vi "dfd_FXP Simu with State.vi"(5 "input range":dbl, 6 "state in":dbl[](array[numeric]) format="%.2f", 7 "input selector":enum16{"FXP", "Integer", "Double"}(ring), 8 "error in (no error)":errorcluster, 9 "filtering statistics in":T3(array[cluster]) {"statistics information"."min value" format="%.2f"; "statistics information"."max value" format="%.2f"; "Quantizer Source" items=["Coefficients a/k"=0, "Coefficients b/v"=7, "Input"=1, "Output"=2, "Multiplicand"=3, "Product"=4, "Sum"=5, "Delay"=6]}, 10 "filter":T4 {"mSRate_QSettings"."source" items=["Coef a/k"=0, "Coef b/v"=7, "Input"=1, "Output"=2, "Multiplicand"=3, "Product"=4, "Sum"=5, "Delay"=6, "Gain"=8]}, 11 "signal in":dbl[](array[numeric])) -> (0 "error out":errorcluster, 1 "filtering statistics out":T3(array[cluster]) {"statistics information"."min value" format="%.2f"; "statistics information"."max value" format="%.2f"; "Quantizer Source" items=["Coefficients a/k"=0, "Coefficients b/v"=7, "Input"=1, "Output"=2, "Multiplicand"=3, "Product"=4, "Sum"=5, "Delay"=6]}, 2 "integer signal out":i32[](array[numeric]), 3 "DBL signal out":dbl[](array[numeric]), 4 "state out":dbl[](array[numeric]) format="%.2f")   [LabVIEW 2017, in "NI_DigFilter_FXP.lvlib"]
uses:
  <vilib>/addons/Digital Filter Design/NI_DigFilter_FXP.lvlib
  <vilib>/addons/Digital Filter Design/_Objects.llb/DFD Filter Obj.ctl
  <vilib>/addons/Digital Filter Design/_Objects.llb/DFD Filter Coef.ctl
  <vilib>/addons/Digital Filter Design/_Objects.llb/DFD Filter Structure Type Selector.ctl
  <vilib>/addons/Digital Filter Design/_Objects.llb/dfd_Internal Quantization Settings.ctl
  <vilib>/addons/Digital Filter Design/_Objects.llb/dfd_Internal Quantization Srcs.ctl
  <vilib>/addons/Digital Filter Design/_Objects.llb/DFD Coef Norm Type.ctl
  <vilib>/addons/Digital Filter Design/_Objects.llb/DFD Quantization Sources.ctl
  <vilib>/addons/Digital Filter Design/_Objects.llb/DFD FXP Statistics Data.ctl
  <vilib>/addons/Digital Filter Design/FXPLib.llb/DFD FXP to I32 (vector).vi
  <vilib>/addons/Digital Filter Design/NI_DigFilterLicensed.lvlib
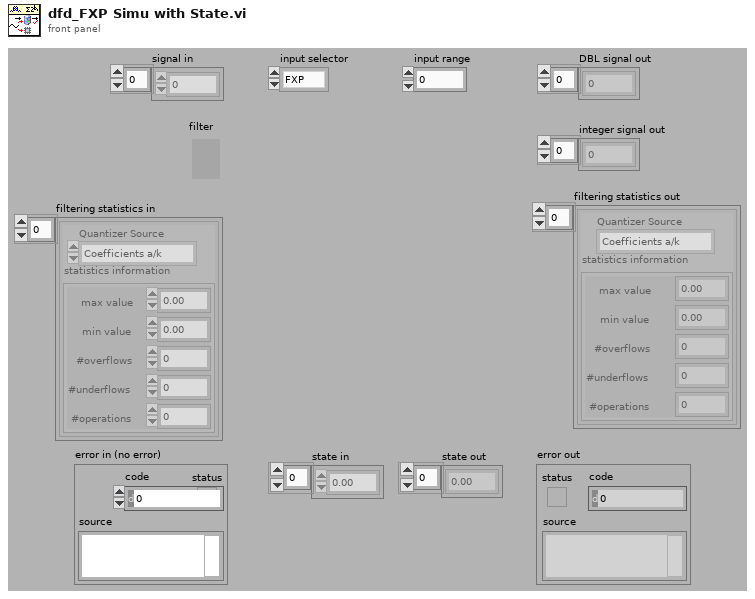
[diagram p1: front panel]
types:
  T1 = typedef "NI_DigFilterLicensed.lvlib/DFD Quantization Sources.ctl" = u16
  T2 = typedef "NI_DigFilterLicensed.lvlib/DFD FXP Statistics Data.ctl" = cluster{"max value":ext, "min value":ext, "#overflows":i32, "#underflows":i32, "#operations":i32}
  T3 = cluster{"Quantizer Source":T1, "statistics information":T2}[]
  T4 = typedef "NI_DigFilterLicensed.lvlib/DFD Filter Obj.ctl" = cluster{"mSRate_Fs":dbl, "mSRate_Version":string, "mSRate_Comments":string, "mSRate_OrgCoef":T5, "mSRate_CurCoef":T5, "mSRate_Quantized?":bool, "mSRate_QCoef":T5, "mSRate_QSettings":T7[], "mSRate_Order":i32, "mSRate_Scaling":cluster{"mSRate_ScaleByPowerOf2?":bool, "mSRate_ScaleType":T9}}
  T5 = typedef "NI_DigFilterLicensed.lvlib/DFD Filter Coef.ctl" = cluster{"type":T6, "gain":dbl, "coef a (k)":dbl[], "coef b (v)":dbl[]}
  T6 = typedef "NI_DigFilterLicensed.lvlib/DFD Filter Structure Type Selector.ctl" = enum16{"Undefined", "FIR Direct Form", "FIR Direct Form Transposed", "FIR Symmetric", "FIR Antisymmetric", "IIR Direct Form I", "IIR Direct Form I Transposed", "IIR Direct Form II", "IIR Direct Form II Transposed", "IIR Cascaded Second Order Sections Form I", "IIR Cascaded Second Order Sections Form I Transposed", "IIR Cascaded Second Order Sections Form II", "IIR Cascaded Second Order Sections Form II Transposed", "Lattice Allpass (basic sections)", "Lattice Allpass (one multiplier sections)", "Lattice Allpass (normalized sections)", "Lattice AR (basic sections)", "Lattice AR (one multiplier sections)", "Lattice AR (normalized sections)", "Lattice MA (minimum phase)", "Lattice MA (maximum phase)", "Lattice ARMA (basic sections)", "Lattice ARMA (one multiplier sections)", "Lattice ARMA (normalized sections)"}
  T7 = typedef "NI_DigFilterLicensed.lvlib/dfd_Internal Quantization Settings.ctl" = cluster{"source":T8, "wl":i16, "iwl":i16, "overflow mode":enum16{"Saturation", "Wrap"}, "rounding mode":enum16{"Nearest", "Truncation"}, "signed?":bool}
  T8 = typedef "NI_DigFilterLicensed.lvlib/dfd_Internal Quantization Srcs.ctl" = u16
  T9 = typedef "NI_DigFilterLicensed.lvlib/DFD Coef Norm Type.ctl" = enum16{"No Norm", "Time Domain 1-Norm", "Time Domain 2-Norm", "Time Domain Inf-Norm"}
  T10 = typedef "dfd_DFXP Operation Parameter.ctl" = cluster{"source":T8, "is floating?":bool, "o-mode":enum16{"Saturation", "Wrap"}, "q-mode":enum16{"Nearest", "Truncation"}, "wl":i16, "high limit":i64, "low limit":i64, "iwl":i16, "sign?":bool}
  T11 = typedef "dfd_DFXP Data Type (vector).ctl" = cluster{"Values":i64[], "wl":i16, "iwl":i16}
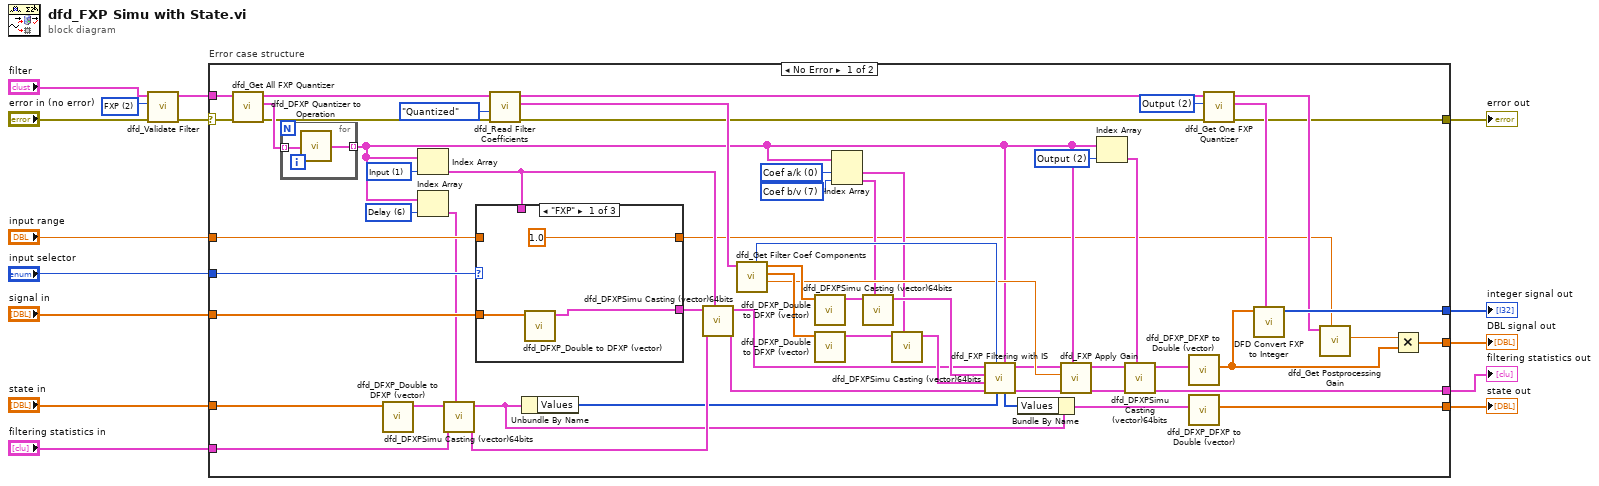
[diagram p0: block diagram]
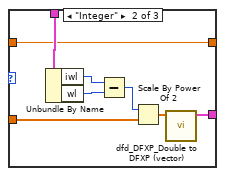
[diagram p2: hidden frame]
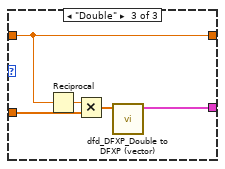
[diagram p3: hidden frame]
diagram:
  w15 = u16 2 items=["Auto", "FLP Only", "FXP"] ("check option")
  n1 = call <vilib>:"dfd_Validate Filter.vi"("error in (no error)"="error in (no error)", "check option"=w15, "filter in"="filter") -> ("error out"=w3:errorcluster, "filter out"=w4:T4)  [unwired: 7 out]
  n2 = case "Error case structure" shown="No Error" w3 {
    selector: w3 -> [w21 w92]
    tunnel: [w68 _] -> w7
    tunnel: [w67 _] -> w6
    tunnel: "signal in" -> [w39 _]
    tunnel: [w41 _] -> w5
    tunnel: w4 -> [w61 _]
    tunnel: "input range" -> [w40 _]
    tunnel: "input selector" -> [w38 _]
    tunnel: "state in" -> [w32 w93]
    tunnel: "filtering statistics in" -> [w28 _]
    tunnel: [w22 w93] -> w8
    tunnel: [w18 w92] -> w1
    frame No Error {
      w31 = T8 6 items=["Coef a/k"=0, "Coef b/v"=7, "Input"=1, "Output"=2, "Multiplicand"=3, "Product"=4, "Sum"=5, "Delay"=6, "Gain"=8] ("quantization source")
      w46 = T8 7 items=["Coef a/k"=0, "Coef b/v"=7, "Input"=1, "Output"=2, "Multiplicand"=3, "Product"=4, "Sum"=5, "Delay"=6, "Gain"=8] ("source")
      w47 = T8 0 items=["Coef a/k"=0, "Coef b/v"=7, "Input"=1, "Output"=2, "Multiplicand"=3, "Product"=4, "Sum"=5, "Delay"=6, "Gain"=8] ("source")
      w55 = T8 2 items=["Coef a/k"=0, "Coef b/v"=7, "Input"=1, "Output"=2, "Multiplicand"=3, "Product"=4, "Sum"=5, "Delay"=6, "Gain"=8] ("quantization source")
      w60 = T8 1 items=["Coef a/k"=0, "Coef b/v"=7, "Input"=1, "Output"=2, "Multiplicand"=3, "Product"=4, "Sum"=5, "Delay"=6, "Gain"=8] ("source")
      w57 = T8 2 items=["Coef a/k"=0, "Coef b/v"=7, "Input"=1, "Output"=2, "Multiplicand"=3, "Product"=4, "Sum"=5, "Delay"=6, "Gain"=8] ("quantization source")
      n3 = call <vilib>:"dfd_Get All FXP Quantizer.vi"("error in (no error)"=w21, "filter in"=w61) -> ("error out"=w20:errorcluster, "quantization settings"=w54:T7[], "filter out"=w59:T4)  [unwired: 7 out]
      n4 = for {
        tunnel: w54 -> [w91] mode=indexing
        tunnel: [w90] -> w30 mode=indexing
        n5 = call <vilib>:"dfd_DFXP Quantizer to Operation.vi"("quantizer"=w91) -> ("op params"=w90:T10)
      }
      n6 = call <vilib>:"dfd_DFXP_Double to DFXP (vector).vi"("value in"=w32) -> ("value out"=w33:T11)  [unwired: 10 out]
      n7 = Index Array(array=w30, index=w60) -> (element=w36:T10)
      n8 = Index Array(array=w30, index=w31) -> (element=w29:T10)
      n9 = call <vilib>:"dfd_DFXPSimu Casting (vector)64bits.vi"("op params"=w29, "filtering statistics in"=w28, "Value in"=w33) -> ("filtering statistics out"=w27:T3, "Value out"=w24:T11)  [unwired: 1 in, 6 out]
      n10 = case shown="\"FXP\"" w38 {
        tunnel: w36 -> [_ w80 _]
        tunnel: w40 -> [_ w77 w85]
        tunnel: w39 -> [w76 w78 w87]
        tunnel: [w75 w79 w86] -> w37
        tunnel: [1.0 ("input range") w77 w85] -> w16
        frame "FXP" {
          n11 = call <vilib>:"dfd_DFXP_Double to DFXP (vector).vi"("value in"=w76) -> ("value out"=w75:T11)  [unwired: 10 out]
        }
        frame "Integer" {
          n12 = Unbundle By Name(w80) -> ("iwl"=w81:i16, "wl"=w82:i16)
          n13 = Subtract(x=w81, y=w82) -> (x-y=w83:i16)
          n14 = Scale By Power Of 2(n=w83, x=w78) -> (x*2^n=w84:dbl[])
          n15 = call <vilib>:"dfd_DFXP_Double to DFXP (vector).vi"("value in"=w84) -> ("value out"=w79:T11)  [unwired: 10 out]
        }
        frame "Double" {
          n16 = Reciprocal(x=w85) -> (1/x=w88:dbl)
          n17 = Multiply(x=w88, y=w87) -> (x*y=w89:dbl[])
          n18 = call <vilib>:"dfd_DFXP_Double to DFXP (vector).vi"("value in"=w89) -> ("value out"=w86:T11)  [unwired: 10 out]
        }
      }
      n19 = call <vilib>:"dfd_Read Filter Coefficients.vi"("error in (no error)"=w20, "coef source"=enum16{"Original", "Current", "Quantized"}."Quantized", "filter in"=w59) -> ("error out"=w19:errorcluster, "filter coef"=w72:T5, "filter out"=w53:T4)  [unwired: 6 out]
      n20 = Unbundle By Name(w24) -> ("Values"=w26:i64[])
      n21 = call <vilib>:"dfd_DFXPSimu Casting (vector)64bits.vi"("op params"=w36, "filtering statistics in"=w27, "Value in"=w37) -> ("filtering statistics out"=w35:T3, "Value out"=w34:T11)  [unwired: 1 in, 6 out]
      n22 = call <vilib>:"dfd_Get Filter Coef Components.vi"("filter coef"=w72) -> ("gain"=w64:dbl, "coef a (k)"=w65:dbl[], "coef b (v)"=w66:dbl[], "type"=w73:T6)  [unwired: 1 in, 6 out]
      n23 = call <vilib>:"dfd_DFXP_Double to DFXP (vector).vi"("value in"=w66) -> ("value out"=w51:T11)  [unwired: 10 out]
      n24 = call <vilib>:"dfd_DFXP_Double to DFXP (vector).vi"("value in"=w65) -> ("value out"=w49:T11)  [unwired: 10 out]
      n25 = Index Array(array=w30, index #1=w47, index #2=w46) -> (element #1=w45:T10, element #2=w44:T10)
      n26 = call <vilib>:"dfd_DFXPSimu Casting (vector)64bits.vi"("op params"=w44, "Value in"=w51) -> ("Value out"=w50:T11)  [unwired: 2 in, 7 out]
      n27 = call <vilib>:"dfd_DFXPSimu Casting (vector)64bits.vi"("op params"=w45, "Value in"=w49) -> ("Value out"=w48:T11)  [unwired: 2 in, 7 out]
      n28 = call <vilib>:"dfd_FXP Filtering with IS.vi"("FXPOPs"=w30, "state in"=w26, "struct typ"=w73, "filtering statistics in"=w35, "coef a"=w48, "coef b"=w50, "X"=w34) -> ("filtering statistics out"=w70:T3, "filtered X"=w58:T11, "state out"=w25:i64[])  [unwired: 2 out]
      n29 = Bundle By Name(cluster=w24, "Values"=w25) -> (w23:T11)
      n30 = call <vilib>:"dfd_FXP Apply Gain.vi"("FXPOPs"=w30, "filtering statistics in"=w70, "gain"=w64, "before-gain X"=w58) -> ("filtering statistics out"=w69:T3, "after-gain X"=w63:T11)  [unwired: 6 out]
      n31 = Index Array(array=w30, index=w57) -> (element=w56:T10)
      n32 = call <vilib>:"dfd_DFXPSimu Casting (vector)64bits.vi"("op params"=w56, "filtering statistics in"=w69, "Value in"=w63) -> ("filtering statistics out"=w68:T3, "Value out"=w62:T11)  [unwired: 1 in, 6 out]
      n33 = call <vilib>:"dfd_DFXP_DFXP to Double (vector).vi"("Value in"=w62) -> ("DBL"=w42:dbl[])  [unwired: 10 out]
      n34 = call <vilib>:"dfd_DFXP_DFXP to Double (vector).vi"("Value in"=w23) -> ("DBL"=w22:dbl[])  [unwired: 10 out]
      n35 = call <vilib>:"dfd_Get One FXP Quantizer.vi"("error in (no error)"=w19, "quantization source"=w55, "filter in"=w53) -> ("error out"=w18:errorcluster, "quantization settings"=w52:T7, "filter out"=w43:T4)  [unwired: 6 out]
      n36 = call-poly <vilib>:"DFD Convert FXP to Integer.vi"("quantization settings"=w52, "FXP values"=w42) -> ("I32 values"=w67:i32[])  [unwired: 1 in, 8 out]
      n37 = call <vilib>:"dfd_Get Postprocessing Gain.vi"("input range"=w16, "filter"=w43) -> ("DBL gain"=w17:dbl)  [unwired: 9 out]
      n38 = Multiply(x=w17, y=w42) -> (x*y=w41:dbl[])
    }
    frame Error {
    }
  }
  "filtering statistics out" <- w7
  "error out" <- w1
  "DBL signal out" <- w5
  "integer signal out" <- w6
  "state out" <- w8
